vi "OnDoubleClick.vi"(0 "XRef":T10, 1 "Point":T8, 2 "Mouse Mods":T6, 3 "State In":T1) -> (14 "Reply":T4, 15 "Fatal Error Out":T3, 16 "State Out":T1)   [LabVIEW 2015, in "LVJSON.lvlib" / "Get Object Parameters.xnode"]
uses:
  Get Object Parameters.xnode
  <vilib>/XNodeSupport/XNodeXNodeRef.ctl
  <vilib>/XNodeSupport/XNodePoint.ctl
  <vilib>/XNodeSupport/XNodeInt.ctl
  <vilib>/XNodeSupport/XNodeMouseMods.ctl
  <vilib>/XNodeSupport/XNodeBool.ctl
  State.ctl
  Parameter.ctl
  <vilib>/XNodeSupport/XNodeStringArray.ctl
  <vilib>/XNodeSupport/XNodeString.ctl
  <vilib>/XNodeSupport/XNodeErrorCluster.ctl
  Shared/Shared.lvlib
  <vilib>/XNodeSupport/NI_XNodeSupport.lvlib
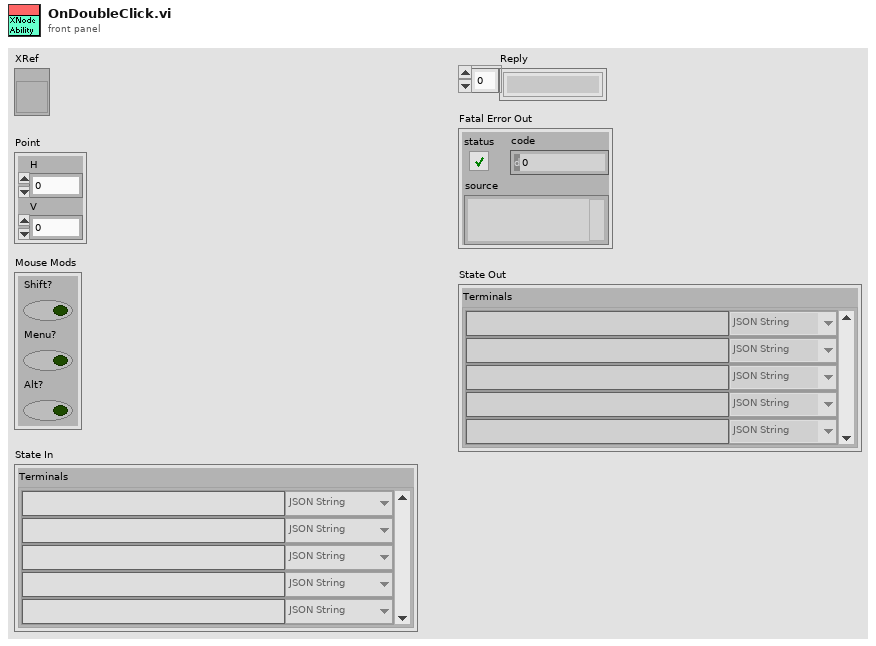
[diagram p1: front panel]
types:
  T1 = typedef "LVJSON.lvlib/Get Object Parameters.xnode/State.ctl" = cluster{"Terminals":T2[]}
  T2 = typedef "LVJSON.lvlib/Shared.lvlib/Parameter.ctl" = cluster{"Parameter Name":string, "JSON Type":enum16{"JSON String", "JSON Numeric", "JSON Boolean", "JSON", "JSON Object", "JSON Array", "String Value", "Numeric Value", "Boolean Value"}}
  T3 = typedef "NI_XNodeSupport.lvlib/XNodeErrorCluster.ctl" = errorcluster
  T4 = typedef "NI_XNodeSupport.lvlib/XNodeStringArray.ctl" = T5[]
  T5 = typedef "NI_XNodeSupport.lvlib/XNodeString.ctl" = string
  T6 = typedef "NI_XNodeSupport.lvlib/XNodeMouseMods.ctl" = cluster{"Shift?":T7, "Menu?":T7, "Alt?":T7}
  T7 = typedef "NI_XNodeSupport.lvlib/XNodeBool.ctl" = bool
  T8 = typedef "NI_XNodeSupport.lvlib/XNodePoint.ctl" = cluster{"H":T9, "V":T9}
  T9 = typedef "NI_XNodeSupport.lvlib/XNodeInt.ctl" = i32
  T10 = typedef "NI_XNodeSupport.lvlib/XNodeXNodeRef.ctl" = refnum<vi>
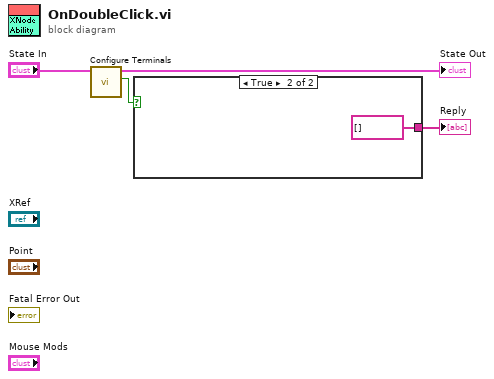
[diagram p0: block diagram]
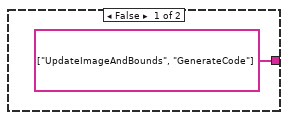
[diagram p2: hidden frame]
diagram:
  n1 = call "Configure Terminals.vi"("State in"="State In") -> ("cancelled?"=w2:bool, "State out"=→"State Out":T1)  [unwired: 9 in]
  n2 = case shown="True" w2 {
    tunnel: [T4 ["UpdateImageAndBounds", "GenerateCode"] ("Reply") T4 [] ("Reply")] -> w1
    frame False {
    }
    frame True {
    }
  }
  "Reply" <- w1
